vi "mobileye_decoder_PC.vi"(8 "can cluster":T1 {"identifier" format="%03x"}, 11 "name":string="Mobileye560") -> ()   [LabVIEW 2015]
uses:
  G_SEN.vi
  G_ALL.vi
panel:
  out "lane both":bool
  out "lane_left":dbl[](array[numeric])
  out "lane_right":dbl[](array[numeric])
  out "next lane left":dbl[][](array[numeric])
  out "next lane right":dbl[][](array[numeric])
  out "obs_tmp":dbl[][](array[numeric])
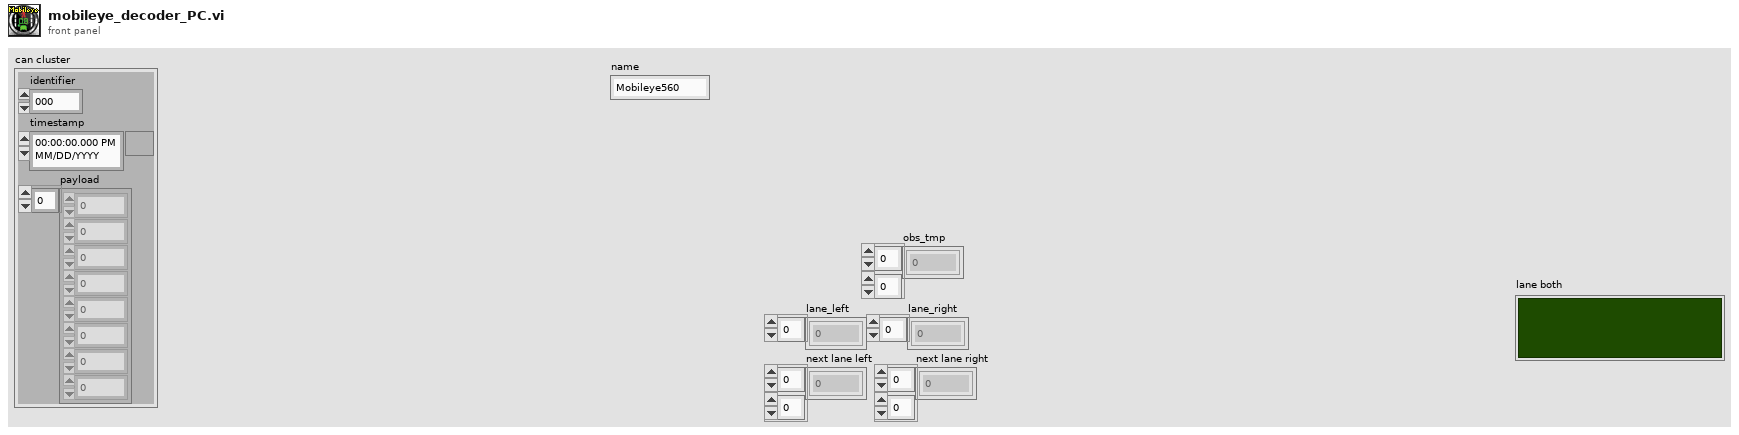
[diagram p1: front panel]
types:
  T1 = cluster{"identifier":u32, "timestamp":timestamp, "payload":u8[]}
  T2 = cluster{"C_Wheel base":dbl, "ratio_steer":dbl, "Overall width":dbl, "af":dbl, "turn radius":dbl, "eval":dbl, "ap":dbl, "an":dbl, "Vmax":dbl, "mu":dbl, "Vlast":dbl}
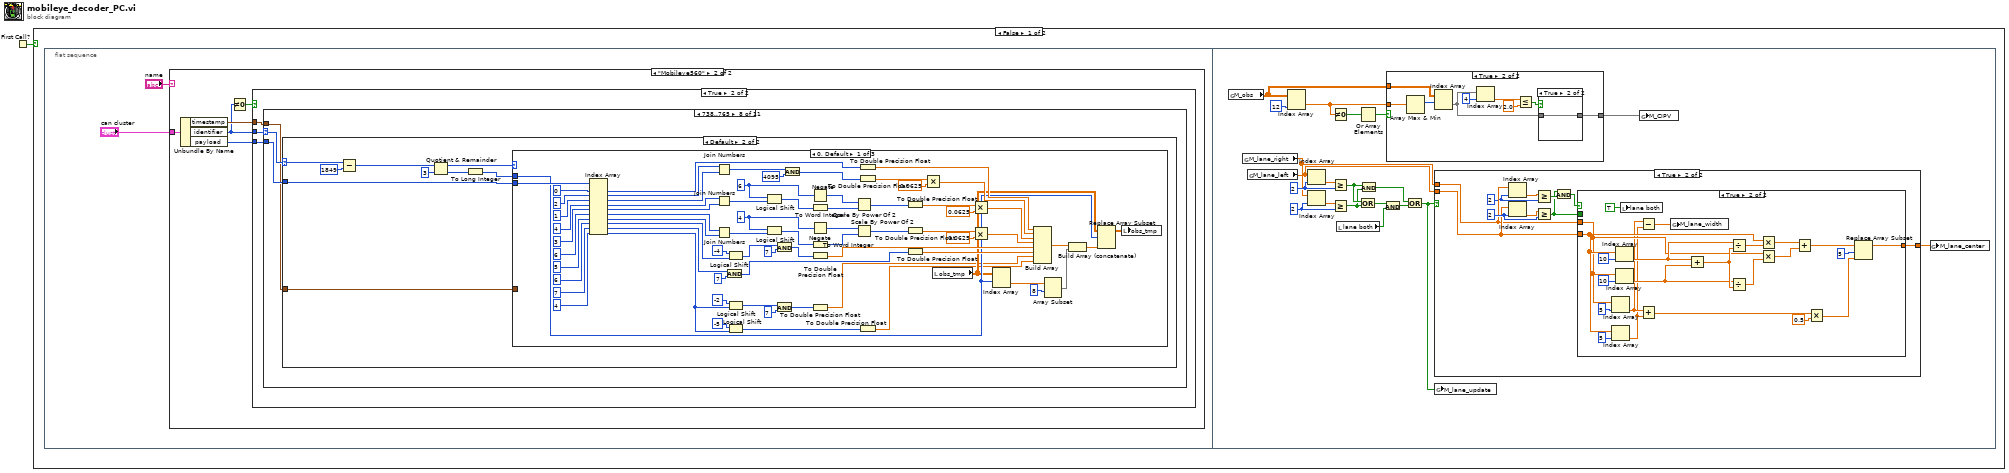
[diagram p0: block diagram]
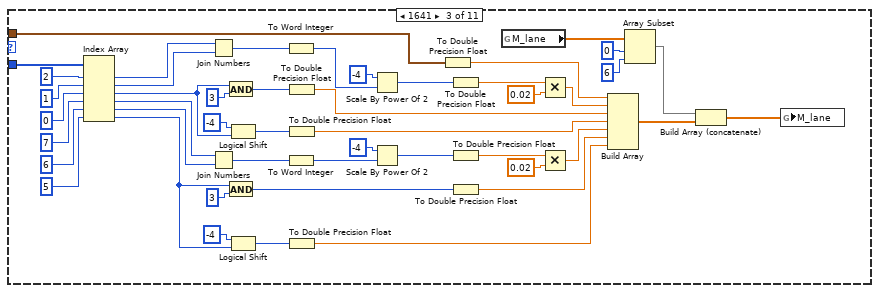
[diagram p6: hidden frame]
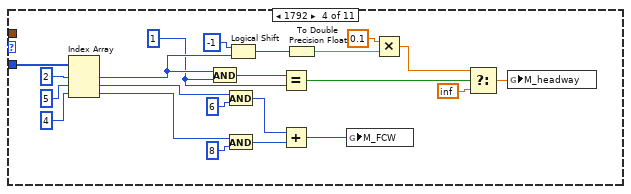
[diagram p7: hidden frame]
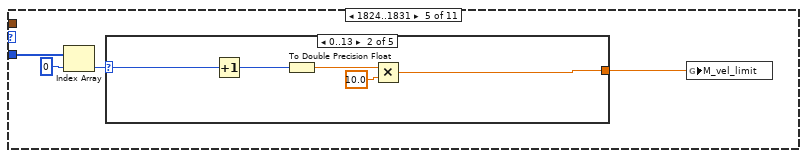
[diagram p8: hidden frame]
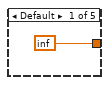
[diagram p9: hidden frame]
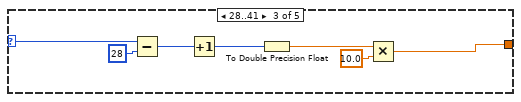
[diagram p10: hidden frame]
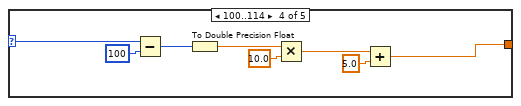
[diagram p11: hidden frame]
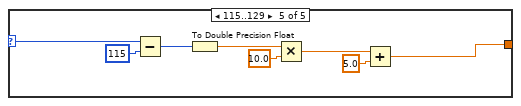
[diagram p12: hidden frame]
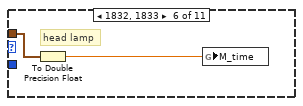
[diagram p13: hidden frame]
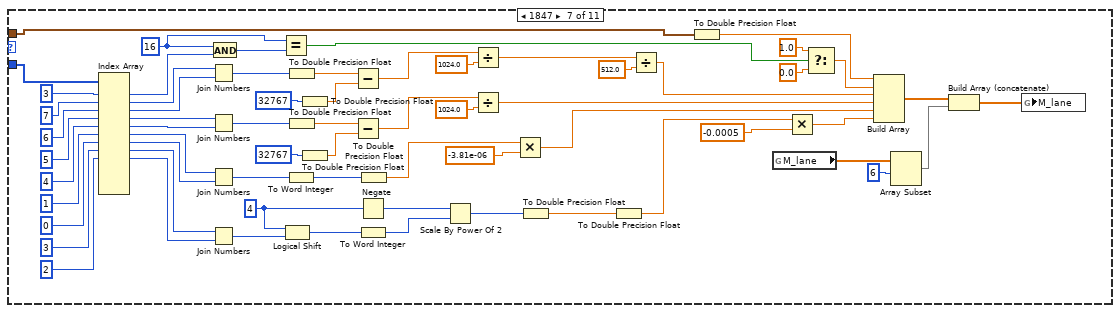
[diagram p14: hidden frame]
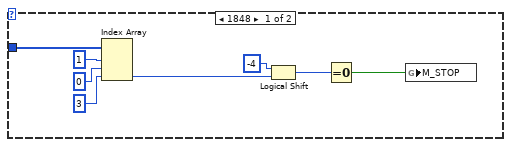
[diagram p15: hidden frame]
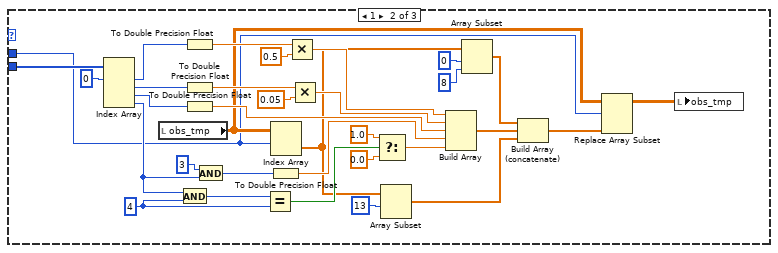
[diagram p16: hidden frame]
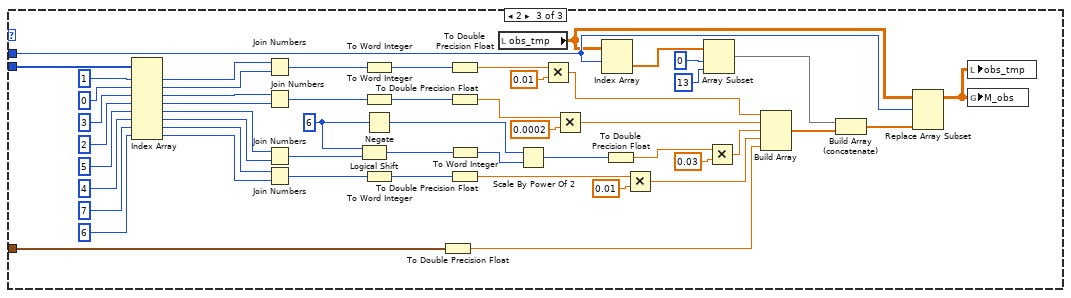
[diagram p17: hidden frame]
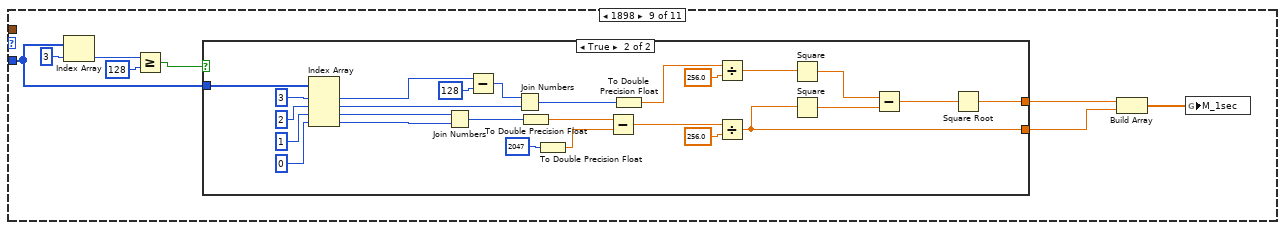
[diagram p18: hidden frame]
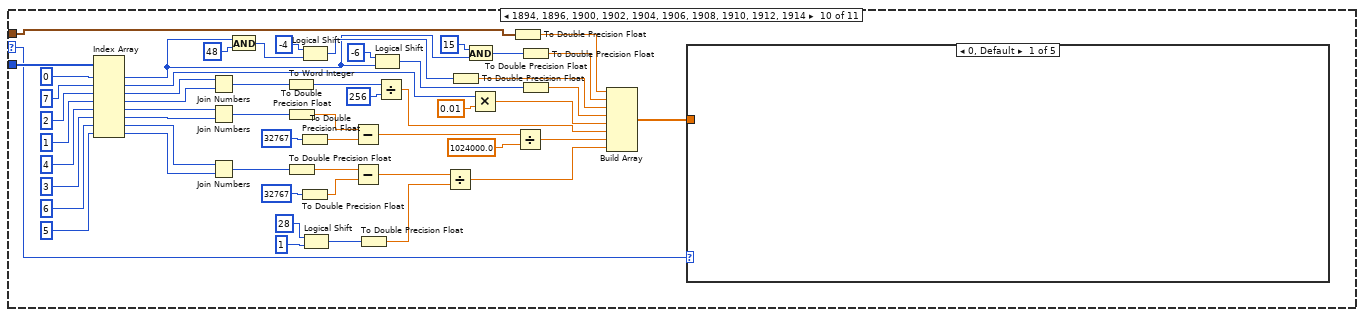
[diagram p20: hidden frame]
diagram:
  n1 = First Call?() -> (First Call?: T/F=w1:bool)
  n2 = case shown="False" w1 {
    frame False {
      n3 = flat-sequence {
        frame #0 {
          n4 = case shown="\"Mobileye560\"" "name" {
            tunnel: "can cluster" -> [_ w8]
            frame "False", Default {
            }
            frame "Mobileye560" {
              n5 = Unbundle By Name(w8) -> ("timestamp"=w6:timestamp, "identifier"=w5:u32, "payload"=w7:u8[])
              n6 = Not Equal To 0?(x=w5) -> (x != 0?=w4:bool)
              n7 = case shown="True" w4 {
                tunnel: w7 -> [_ w11]
                tunnel: w6 -> [_ w10]
                tunnel: w5 -> [_ w9]
                frame False {
                }
                frame True {
                  n8 = case shown="738..765" w9 {
                    selector: w9 -> [_ _ _ _ _ _ _ w181 _ w388 w469]
                    tunnel: w11 -> [_ _ w58 w80 w84 _ w178 w180 w357 w442 w497]
                    tunnel: w10 -> [_ _ w35 _ _ w115 w122 w179 _ w408 w472]
                    frame 0, Default {
                    }
                    frame 1616 {
                      # "Fixed Yaw horizontal"
                    }
                    frame 1641 {
                      n9 = Index Array(array=w58, index #1=2 ("index"), index #2=1 ("index"), index #3=0 ("index"), index #4=7 ("index"), index #5=6 ("index"), index #6=5 ("index")) -> (element #1=w55:u8, element #2=w54:u8, element #3=w33:u8, element #4=w26:u8, element #5=w25:u8, element #6=w21:u8)
                      n10 = Join Numbers(hi=w55, lo=w54) -> ((hi.lo)=w53:u16)
                      n11 = Join Numbers(hi=w26, lo=w25) -> ((hi.lo)=w48:u16)
                      n12 = And(x=w33, y=u8 3) -> (x .and. y?=w32:u8)
                      n13 = And(x=w21, y=u8 3) -> (x .and. y?=w24:u8)
                      n14 = Logical Shift(y=i16 -4, x=w33) -> (x << y=w31:u8)
                      n15 = Logical Shift(y=i16 -4, x=w21) -> (x << y=w28:u8)
                      n16 = To Word Integer(number=w53) -> (16bit integer=w40:i16)
                      n17 = To Word Integer(number=w48) -> (16bit integer=w37:i16)
                      n18 = To Double Precision Float(number=w32) -> (double precision float=w30:dbl)
                      n19 = To Double Precision Float(number=w31) -> (double precision float=w29:dbl)
                      n20 = To Double Precision Float(number=w28) -> (double precision float=w22:dbl)
                      n21 = Scale By Power Of 2(n=i16 -4 ("y"), x=w40) -> (x*2^n=w39:i16)
                      n22 = Scale By Power Of 2(n=i16 -4 ("y"), x=w37) -> (x*2^n=w36:i16)
                      n23 = To Double Precision Float(number=w35) -> (double precision float=w20:dbl)
                      n24 = To Double Precision Float(number=w39) -> (double precision float=w52:dbl)
                      n25 = To Double Precision Float(number=w36) -> (double precision float=w49:dbl)
                      n26 = To Double Precision Float(number=w24) -> (double precision float=w23:dbl)
                      n27 = global read "G_SEN.vi" "M_lane"() -> (w12:dbl[])
                      n28 = Multiply(x=w52, y=0.02) -> (x*y=w15:dbl)
                      n29 = Multiply(x=w49, y=0.02) -> (x*y=w14:dbl)
                      n30 = Build Array(w20, w15, w30, w29, w14, w23, w22) -> (w16:dbl[])
                      n31 = Array Subset(array=w12, index=0, length=6) -> (w17:dbl[])
                      n32 = Build Array (concatenate)(w17, w16) -> (w13:dbl[])
                      n33 = global write "G_SEN.vi" "M_lane"(w13) -> ()
                    }
                    frame 1792 {
                      w75 = u8 1 ("y")
                      n34 = Index Array(array=w80, index #1=2 ("index"), index #2=5 ("index"), index #3=4 ("index")) -> (element #1=w78:u8, element #2=w67:u8, element #3=w63:u8)
                      n35 = And(x=w78, y=w75) -> (x .and. y?=w76:u8)
                      n36 = And(x=w67, y=u8 6) -> (x .and. y?=w62:u8)
                      n37 = And(x=w63, y=u8 8) -> (x .and. y?=w61:u8)
                      n38 = Logical Shift(y=i16 -1, x=w78) -> (x << y=w73:u8)
                      n39 = Equal?(x=w76, y=w75) -> (x = y?=w74:bool)
                      n40 = Add(x=w62, y=w61) -> (x+y=w60:u8)
                      n41 = To Double Precision Float(number=w73) -> (double precision float=w72:dbl)
                      n42 = global write "G_SEN.vi" "M_FCW"(w60) -> ()
                      n43 = Multiply(x=0.1, y=w72) -> (x*y=w70:dbl)
                      n44 = Select(t=w70, s=w74, f=inf) -> (s? t:f=w59:dbl)
                      n45 = global write "G_SEN.vi" "M_headway"(w59) -> ()
                    }
                    frame 1824..1831 {
                      n46 = Index Array(array=w84, index=0) -> (element=w82:u8)
                      n47 = case shown="0..13" w82 {
                        selector: w82 -> [_ w90 w93 w103 w111]
                        tunnel: [inf w86 w94 w98 w106] -> w81
                        frame Default {
                        }
                        frame 0..13 {
                          n48 = Increment(x=w90) -> (x+1=w89:u8)
                          n49 = To Double Precision Float(number=w89) -> (double precision float=w88:dbl)
                          n50 = Multiply(x=w88, y=10.0) -> (x*y=w86:dbl)
                        }
                        frame 28..41 {
                          n51 = Subtract(x=w93, y=u8 28) -> (x-y=w92:u8)
                          n52 = Increment(x=w92) -> (x+1=w97:u8)
                          n53 = To Double Precision Float(number=w97) -> (double precision float=w96:dbl)
                          n54 = Multiply(x=w96, y=10.0) -> (x*y=w94:dbl)
                        }
                        frame 100..114 {
                          n55 = Subtract(x=w103, y=u8 100) -> (x-y=w101:u8)
                          n56 = To Double Precision Float(number=w101) -> (double precision float=w105:dbl)
                          n57 = Multiply(x=w105, y=10.0) -> (x*y=w100:dbl)
                          n58 = Add(x=w100, y=5.0) -> (x+y=w98:dbl)
                        }
                        frame 115..129 {
                          n59 = Subtract(x=w111, y=u8 115) -> (x-y=w109:u8)
                          n60 = To Double Precision Float(number=w109) -> (double precision float=w113:dbl)
                          n61 = Multiply(x=w113, y=10.0) -> (x*y=w108:dbl)
                          n62 = Add(x=w108, y=5.0) -> (x+y=w106:dbl)
                        }
                      }
                      n63 = global write "G_SEN.vi" "M_vel_limit"(w81) -> ()
                    }
                    frame 1832, 1833 {
                      # "head lamp"
                      n64 = To Double Precision Float(number=w115) -> (double precision float=w114:dbl)
                      n65 = global write "G_SEN.vi" "M_time"(w114) -> ()
                    }
                    frame 1847 {
                      w155 = u8 16 ("x")
                      w157 = i16 4 ("x")
                      n66 = Index Array(array=w178, index #1=3 ("index"), index #2=7 ("index"), index #3=6 ("index"), index #4=5 ("index"), index #5=4 ("index"), index #6=1 ("index"), index #7=0 ("index"), index #8=3 ("index"), index #9=2 ("index")) -> (element #1=w138:u8, element #2=w132:u8, element #3=w131:u8, element #4=w130:u8, element #5=w129:u8, element #6=w175:u8, element #7=w174:u8, element #8=w167:u8, element #9=w166:u8)  [unwired: 4 in, 4 out]
                      n67 = Join Numbers(hi=w132, lo=w131) -> ((hi.lo)=w154:u16)
                      n68 = Join Numbers(hi=w130, lo=w129) -> ((hi.lo)=w142:u16)
                      n69 = Join Numbers(hi=w175, lo=w174) -> ((hi.lo)=w173:u16)
                      n70 = Join Numbers(hi=w167, lo=w166) -> ((hi.lo)=w161:u16)
                      n71 = And(x=w155, y=w138) -> (x .and. y?=w156:u8)
                      n72 = Equal?(x=w155, y=w156) -> (x = y?=w141:bool)
                      n73 = Logical Shift(y=w157, x=w161) -> (x << y=w165:u16)
                      n74 = To Word Integer(number=w173) -> (16bit integer=w172:i16)
                      n75 = To Double Precision Float(number=w154) -> (double precision float=w153:dbl)
                      n76 = To Double Precision Float(number=w142) -> (double precision float=w143:dbl)
                      n77 = To Double Precision Float(number=i16 32767) -> (double precision float=w151:dbl)
                      n78 = To Double Precision Float(number=i16 32767) -> (double precision float=w145:dbl)
                      n79 = Subtract(x=w153, y=w151) -> (x-y=w150:dbl)
                      n80 = Subtract(x=w143, y=w145) -> (x-y=w146:dbl)
                      n81 = Negate(x=w157) -> (-x=w160:i16)
                      n82 = To Word Integer(number=w165) -> (16bit integer=w159:i16)
                      n83 = To Double Precision Float(number=w172) -> (double precision float=w171:dbl)
                      n84 = Scale By Power Of 2(n=w160, x=w159) -> (x*2^n=w158:i16)
                      n85 = Divide(x=w150, y=1024.0) -> (x/y=w127:dbl)
                      n86 = Divide(x=w146, y=1024.0) -> (x/y=w125:dbl)
                      n87 = Multiply(x=w171, y=-3.81e-06) -> (x*y=w124:dbl)
                      n88 = To Double Precision Float(number=w158) -> (double precision float=w162:dbl)
                      n89 = To Double Precision Float(number=w162) -> (double precision float=w163:dbl)
                      n90 = Divide(x=w127, y=512.0) -> (x/y=w126:dbl)
                      n91 = To Double Precision Float(number=w122) -> (double precision float=w118:dbl)
                      n92 = global read "G_SEN.vi" "M_lane"() -> (w116:dbl[])
                      n93 = Multiply(x=w163, y=-0.0005) -> (x*y=w123:dbl)
                      n94 = Select(t=1.0, s=w141, f=0.0) -> (s? t:f=w128:dbl)
                      n95 = Build Array(w118, w128, w126, w125, w124, w123) -> (w120:dbl[])
                      n96 = Array Subset(array=w116, index=6) -> (w119:dbl[])  [unwired: 1 in]
                      n97 = Build Array (concatenate)(w120, w119) -> (w117:dbl[])
                      n98 = global write "G_SEN.vi" "M_lane"(w117) -> ()
                    }
                    frame 1848..1893 {
                      n99 = case shown="Default" w181 {
                        selector: w181 -> [_ w194]
                        tunnel: w180 -> [w189 w193]
                        tunnel: w179 -> [_ w190]
                        frame 1848 {
                          n100 = Index Array(array=w189, index #1=1 ("index"), index #2=0 ("index"), index #3=3 ("index")) -> (element #3=w184:u8)  [unwired: 2 out]
                          n101 = Logical Shift(y=i16 -4, x=w184) -> (x << y=w186:u8)
                          n102 = Equal To 0?(x=w186) -> (x = 0?=w182:bool)
                          n103 = global write "G_SEN.vi" "M_STOP"(w182) -> ()
                        }
                        frame Default {
                          n104 = Subtract(x=w194, y=u32 1849) -> (x-y=w197:u32)
                          n105 = Quotient & Remainder(x=w197, y=u32 3) -> (x-y*floor(x/y)=w195:u32, floor(x/y)=w192:u32)
                          n106 = To Long Integer(number=w192) -> (32bit integer=w191:i32)
                          n107 = case shown="0, Default" w195 {
                            tunnel: w193 -> [w268 w301 w353]
                            tunnel: w191 -> [w222 w276 w352]
                            tunnel: w190 -> [_ _ w304]
                            frame 0, Default {
                              w211 = i16 4 ("y")
                              w215 = i16 6 ("y")
                              n108 = Index Array(array=w268, index #1=0 ("index"), index #2=2 ("index"), index #3=1 ("index"), index #4=4 ("index"), index #5=3 ("index"), index #6=6 ("index"), index #7=5 ("index"), index #8=6 ("index"), index #9=7 ("index"), index #10=4 ("index")) -> (element #1=w260:u8, element #2=w264:u8, element #3=w263:u8, element #4=w252:u8, element #5=w251:u8, element #6=w239:u8, element #7=w238:u8, element #8=w234:u8, element #9=w227:u8, element #10=w201:u8)
                              n109 = Join Numbers(hi=w264, lo=w263) -> ((hi.lo)=w255:u16)
                              n110 = Join Numbers(hi=w252, lo=w251) -> ((hi.lo)=w250:u16)
                              n111 = Join Numbers(hi=w239, lo=w238) -> ((hi.lo)=w240:u16)
                              n112 = And(x=w227, y=u8 7) -> (x .and. y?=w226:u8)
                              n113 = Logical Shift(y=i16 -4, x=w234) -> (x << y=w233:u8)
                              n114 = Logical Shift(y=i16 -2, x=w201) -> (x << y=w203:u8)
                              n115 = Logical Shift(y=i16 -5, x=w201) -> (x << y=w207:u8)
                              n116 = Logical Shift(y=w215, x=w250) -> (x << y=w249:u16)
                              n117 = Logical Shift(y=w211, x=w240) -> (x << y=w241:u16)
                              n118 = And(x=w233, y=u8 7) -> (x .and. y?=w231:u8)
                              n119 = And(x=w203, y=u8 7) -> (x .and. y?=w205:u8)
                              n120 = And(x=w255, y=u16 4095) -> (x .and. y?=w261:u16)
                              n121 = Negate(x=w215) -> (-x=w216:i16)
                              n122 = To Word Integer(number=w249) -> (16bit integer=w214:i16)
                              n123 = Negate(x=w211) -> (-x=w212:i16)
                              n124 = To Word Integer(number=w241) -> (16bit integer=w210:i16)
                              n125 = To Double Precision Float(number=w231) -> (double precision float=w230:dbl)
                              n126 = To Double Precision Float(number=w205) -> (double precision float=w200:dbl)
                              n127 = Scale By Power Of 2(n=w216, x=w214) -> (x*2^n=w213:i16)
                              n128 = Scale By Power Of 2(n=w212, x=w210) -> (x*2^n=w209:i16)
                              n129 = To Double Precision Float(number=w260) -> (double precision float=w257:dbl)
                              n130 = To Double Precision Float(number=w261) -> (double precision float=w259:dbl)
                              n131 = To Double Precision Float(number=w207) -> (double precision float=w199:dbl)
                              n132 = To Double Precision Float(number=w213) -> (double precision float=w246:dbl)
                              n133 = To Double Precision Float(number=w209) -> (double precision float=w243:dbl)
                              n134 = To Double Precision Float(number=w226) -> (double precision float=w225:dbl)
                              n135 = Multiply(x=w259, y=0.0625) -> (x*y=w256:dbl)
                              n136 = local read "obs_tmp"() -> (w221:dbl[][])
                              n137 = Multiply(x=w246, y=0.0625) -> (x*y=w247:dbl)
                              n138 = Multiply(x=w243, y=0.0625) -> (x*y=w237:dbl)
                              n139 = Index Array(array=w221, index (row)=w222) -> (element=w219:dbl[])  [unwired: 1 in]
                              n140 = Build Array(w257, w256, w247, w237, w230, w225, w200, w199) -> (w224:dbl[])
                              n141 = Array Subset(array=w219, index=8) -> (w218:dbl[])  [unwired: 1 in]
                              n142 = Build Array (concatenate)(w224, w218) -> (w223:dbl[])
                              n143 = Replace Array Subset(array=w221, new element=w223, index (row)=w222) -> (w220:dbl[][])  [unwired: 1 in]
                              n144 = local write "obs_tmp"(w220) -> ()
                            }
                            frame 1 {
                              w286 = u8 4 ("y")
                              n145 = Index Array(array=w301, index #1=0 ("index")) -> (element #1=w299:u8, element #2=w293:u8, element #3=w291:u8, element #4=w280:u8)  [unwired: 3 in]
                              n146 = local read "obs_tmp"() -> (w278:dbl[][])
                              n147 = And(x=w280, y=w286) -> (x .and. y?=w287:u8)
                              n148 = To Double Precision Float(number=w299) -> (double precision float=w298:dbl)
                              n149 = To Double Precision Float(number=w293) -> (double precision float=w294:dbl)
                              n150 = To Double Precision Float(number=w291) -> (double precision float=w290:dbl)
                              n151 = And(x=u8 3 ("y"), y=w280) -> (x .and. y?=w289:u8)
                              n152 = Equal?(x=w287, y=w286) -> (x = y?=w285:bool)
                              n153 = Index Array(array=w278, index (row)=w276) -> (element=w273:dbl[])  [unwired: 1 in]
                              n154 = To Double Precision Float(number=w289) -> (double precision float=w288:dbl)
                              n155 = Multiply(x=w298, y=0.5) -> (x*y=w296:dbl)
                              n156 = Multiply(x=w294, y=0.05) -> (x*y=w292:dbl)
                              n157 = Select(t=1.0, s=w285, f=0.0) -> (s? t:f=w282:dbl)
                              n158 = Array Subset(array=w273, index=13) -> (w269:dbl[])  [unwired: 1 in]
                              n159 = Build Array(w296, w292, w290, w288, w282) -> (w270:dbl[])
                              n160 = Array Subset(array=w273, index=0, length=8) -> (w271:dbl[])
                              n161 = Build Array (concatenate)(w271, w270, w269) -> (w279:dbl[])
                              n162 = Replace Array Subset(array=w278, new element=w279, index (row)=w276) -> (w277:dbl[][])  [unwired: 1 in]
                              n163 = local write "obs_tmp"(w277) -> ()
                            }
                            frame 2 {
                              w326 = i16 6 ("y")
                              n164 = Index Array(array=w353, index #1=1 ("index"), index #2=0 ("index"), index #3=3 ("index"), index #4=2 ("index"), index #5=5 ("index"), index #6=4 ("index"), index #7=7 ("index"), index #8=6 ("index")) -> (element #1=w349:u8, element #2=w348:u8, element #3=w336:u8, element #4=w335:u8, element #5=w331:u8, element #6=w330:u8, element #7=w314:u8, element #8=w313:u8)
                              n165 = Join Numbers(hi=w349, lo=w348) -> ((hi.lo)=w347:u16)
                              n166 = Join Numbers(hi=w336, lo=w335) -> ((hi.lo)=w337:u16)
                              n167 = Join Numbers(hi=w331, lo=w330) -> ((hi.lo)=w329:u16)
                              n168 = Join Numbers(hi=w314, lo=w313) -> ((hi.lo)=w315:u16)
                              n169 = Logical Shift(y=w326, x=w329) -> (x << y=w328:u16)
                              n170 = To Word Integer(number=w347) -> (16bit integer=w346:i16)
                              n171 = To Word Integer(number=w337) -> (16bit integer=w338:i16)
                              n172 = Negate(x=w326) -> (-x=w327:i16)
                              n173 = To Word Integer(number=w315) -> (16bit integer=w316:i16)
                              n174 = To Double Precision Float(number=w304) -> (double precision float=w303:dbl)
                              n175 = To Double Precision Float(number=w346) -> (double precision float=w345:dbl)
                              n176 = To Double Precision Float(number=w338) -> (double precision float=w339:dbl)
                              n177 = To Word Integer(number=w328) -> (16bit integer=w325:i16)
                              n178 = To Double Precision Float(number=w316) -> (double precision float=w317:dbl)
                              n179 = local read "obs_tmp"() -> (w311:dbl[][])
                              n180 = Scale By Power Of 2(n=w327, x=w325) -> (x*2^n=w324:i16)
                              n181 = Multiply(x=w345, y=0.01) -> (x*y=w343:dbl)
                              n182 = Multiply(x=w339, y=0.0002) -> (x*y=w334:dbl)
                              n183 = Index Array(array=w311, index (row)=w352) -> (element=w308:dbl[])  [unwired: 1 in]
                              n184 = To Double Precision Float(number=w324) -> (double precision float=w322:dbl)
                              n185 = Multiply(x=w317, y=0.01) -> (x*y=w312:dbl)
                              n186 = Array Subset(array=w308, index=0, length=13) -> (w305:dbl[])
                              n187 = Multiply(x=w322, y=0.03) -> (x*y=w321:dbl)
                              n188 = Build Array(w343, w334, w321, w312, w303) -> (w307:dbl[])
                              n189 = Build Array (concatenate)(w305, w307) -> (w306:dbl[])
                              n190 = Replace Array Subset(array=w311, new element=w306, index (row)=w352) -> (w302:dbl[][])  [unwired: 1 in]
                              n191 = local write "obs_tmp"(w302) -> ()
                              n192 = global write "G_SEN.vi" "M_obs"(w302) -> ()
                            }
                          }
                        }
                      }
                    }
                    frame 1898 {
                      n193 = Index Array(array=w357, index=3) -> (element=w360:u8)
                      n194 = Greater Or Equal?(x=w360, y=u8 128) -> (x >= y?=w358:bool)
                      n195 = case shown="True" w358 {
                        tunnel: w357 -> [_ w387]
                        tunnel: [_ w362] -> w356
                        tunnel: [_ w364] -> w355
                        frame False {
                        }
                        frame True {
                          n196 = Index Array(array=w387, index #1=3 ("index"), index #2=2 ("index"), index #3=1 ("index"), index #4=0 ("index")) -> (element #1=w378:u8, element #2=w382:u8, element #3=w381:u8, element #4=w380:u8)
                          n197 = Join Numbers(hi=w381, lo=w380) -> ((hi.lo)=w368:u16)
                          n198 = Subtract(x=w378, y=u8 128) -> (x-y=w377:u8)
                          n199 = Join Numbers(hi=w377, lo=w382) -> ((hi.lo)=w370:u16)
                          n200 = To Double Precision Float(number=w368) -> (double precision float=w376:dbl)
                          n201 = To Double Precision Float(number=u16 2047 ("(hi.lo)")) -> (double precision float=w375:dbl)
                          n202 = Subtract(x=w376, y=w375) -> (x-y=w373:dbl)
                          n203 = To Double Precision Float(number=w370) -> (double precision float=w369:dbl)
                          n204 = Divide(x=w369, y=256.0) -> (x/y=w367:dbl)
                          n205 = Divide(x=w373, y=256.0) -> (x/y=w364:dbl)
                          n206 = Square(x=w367) -> (x^2=w366:dbl)
                          n207 = Square(x=w364) -> (x^2=w365:dbl)
                          n208 = Subtract(x=w366, y=w365) -> (x-y=w363:dbl)
                          n209 = Square Root(x=w363) -> (sqrt(x)=w362:dbl)
                        }
                      }
                      n210 = Build Array(w356, w355) -> (w354:dbl[])
                      n211 = global write "G_SEN.vi" "M_1sec"(w354) -> ()
                    }
                    frame 1894, 1896, 1900, 1902, 1904, 1906, 1908, 1910, 1912, 1914 {
                      n212 = Index Array(array=w442, index #1=0 ("index"), index #2=7 ("index"), index #3=2 ("index"), index #4=1 ("index"), index #5=4 ("index"), index #6=3 ("index"), index #7=6 ("index"), index #8=5 ("index")) -> (element #1=w398:u8, element #2=w393:u8, element #3=w440:u8, element #4=w439:u8, element #5=w432:u8, element #6=w431:u8, element #7=w422:u8, element #8=w421:u8)
                      n213 = Join Numbers(hi=w440, lo=w439) -> ((hi.lo)=w438:u16)
                      n214 = Join Numbers(hi=w432, lo=w431) -> ((hi.lo)=w430:u16)
                      n215 = Join Numbers(hi=w422, lo=w421) -> ((hi.lo)=w415:u16)
                      n216 = And(x=w398, y=u8 48) -> (x .and. y?=w403:u8)
                      n217 = To Word Integer(number=w438) -> (16bit integer=w437:i16)
                      n218 = To Double Precision Float(number=w430) -> (double precision float=w427:dbl)
                      n219 = To Double Precision Float(number=w415) -> (double precision float=w418:dbl)
                      n220 = Logical Shift(y=i16 -4, x=w403) -> (x << y=w401:u8)
                      n221 = To Double Precision Float(number=u16 32767 ("y")) -> (double precision float=w428:dbl)
                      n222 = To Double Precision Float(number=u16 32767 ("y")) -> (double precision float=w417:dbl)
                      n223 = Logical Shift(y=28, x=1) -> (x << y=w412:i32)
                      n224 = Subtract(x=w427, y=w428) -> (x-y=w426:dbl)
                      n225 = Subtract(x=w418, y=w417) -> (x-y=w410:dbl)
                      n226 = To Double Precision Float(number=w412) -> (double precision float=w411:dbl)
                      n227 = Logical Shift(y=i16 -6, x=w398) -> (x << y=w396:u8)
                      n228 = Divide(x=w437, y=i16 256) -> (x/y=w423:dbl)
                      n229 = Divide(x=w410, y=w411) -> (x/y=w409:dbl)
                      n230 = To Double Precision Float(number=w401) -> (double precision float=w399:dbl)
                      n231 = And(x=u8 15, y=w398) -> (x .and. y?=w405:u8)
                      n232 = Multiply(x=w393, y=0.01) -> (x*y=w391:dbl)
                      n233 = To Double Precision Float(number=w408) -> (double precision float=w390:dbl)
                      n234 = Divide(x=w426, y=1024000.0) -> (x/y=w424:dbl)
                      n235 = To Double Precision Float(number=w405) -> (double precision float=w400:dbl)
                      n236 = To Double Precision Float(number=w396) -> (double precision float=w395:dbl)
                      n237 = Build Array(w390, w400, w399, w395, w391, w423, w424, w409) -> (w389:dbl[])
                      n238 = case shown="0, Default" w388 {
                        selector: w388 -> [_ _ _ w458 w466]
                        tunnel: w389 -> [_ w444 w450 w459 w467]
                        frame 0, Default {
                        }
                        frame 1894 {
                          n239 = local read "lane_left"() -> (w447:dbl[])
                          n240 = Array Subset(array=w447, index=8) -> (w445:dbl[])  [unwired: 1 in]
                          n241 = Build Array (concatenate)(w444, w445) -> (w443:dbl[])
                          n242 = local write "lane_left"(w443) -> ()
                        }
                        frame 1896 {
                          n243 = local read "lane_right"() -> (w452:dbl[])
                          n244 = Array Subset(array=w452, index=8) -> (w449:dbl[])  [unwired: 1 in]
                          n245 = Build Array (concatenate)(w450, w449) -> (w448:dbl[])
                          n246 = local write "lane_right"(w448) -> ()
                        }
                        frame 1900, 1904, 1908, 1912 {
                          n247 = Subtract(x=w458, y=u32 1900) -> (x-y=w456:u32)
                          n248 = Quotient & Remainder(x=w456, y=u32 4) -> (floor(x/y)=w454:u32)  [unwired: 1 out]
                          n249 = local read "next lane left"() -> (w460:dbl[][])
                          n250 = Replace Array Subset(array=w460, new element=w459, index (row)=w454) -> (w453:dbl[][])  [unwired: 1 in]
                          n251 = local write "next lane left"(w453) -> ()
                        }
                        frame 1902, 1906, 1910, 1914 {
                          n252 = Subtract(x=w466, y=u32 1900) -> (x-y=w464:u32)
                          n253 = Quotient & Remainder(x=w464, y=u32 4) -> (floor(x/y)=w462:u32)  [unwired: 1 out]
                          n254 = local read "next lane right"() -> (w468:dbl[][])
                          n255 = Replace Array Subset(array=w468, new element=w467, index (row)=w462) -> (w461:dbl[][])  [unwired: 1 in]
                          n256 = local write "next lane right"(w461) -> ()
                        }
                      }
                    }
                    frame 1895, 1897, 1901, 1903, 1905, 1907, 1909, 1911, 1913, 1915 {
                      w479 = u16 32768 ("y")
                      n257 = Index Array(array=w497, index #1=1 ("index"), index #2=0 ("index"), index #3=3 ("index"), index #4=2 ("index")) -> (element #1=w494:u8, element #2=w493:u8, element #3=w484:u8, element #4=w483:u8)
                      n258 = Join Numbers(hi=w494, lo=w493) -> ((hi.lo)=w489:u16)
                      n259 = Join Numbers(hi=w484, lo=w483) -> ((hi.lo)=w480:u16)
                      n260 = Subtract(x=w480, y=w479) -> (x-y=w478:u16)
                      n261 = And(x=w479, y=w480) -> (x .and. y?=w482:u16)
                      n262 = To Double Precision Float(number=w489) -> (double precision float=w490:dbl)
                      n263 = To Double Precision Float(number=u16 32767 ("y")) -> (double precision float=w491:dbl)
                      n264 = Subtract(x=w490, y=w491) -> (x-y=w488:dbl)
                      n265 = Equal?(x=w479, y=w482) -> (x = y?=w481:bool)
                      n266 = Divide(x=w478, y=u16 256) -> (x/y=w476:dbl)
                      n267 = Select(t=w476, s=w481, f=0.0) -> (s? t:f=w473:dbl)
                      n268 = Divide(x=w488, y=1024.0) -> (x/y=w474:dbl)
                      n269 = To Double Precision Float(number=w472) -> (double precision float=w471:dbl)
                      n270 = Build Array(w471, w474, w473) -> (w470:dbl[])
                      n271 = case shown="767" w469 {
                        selector: w469 -> [_ _ _ w519 w534]
                        tunnel: w470 -> [_ w499 w505 w515 w530]
                        frame 0, Default {
                        }
                        frame 1895 {
                          n272 = local read "lane_left"() -> (w503:dbl[])
                          n273 = Array Subset(array=w503, index=0, length=8 ("index")) -> (w502:dbl[])
                          n274 = Build Array (concatenate)(w502, w499) -> (w498:dbl[])
                          n275 = local write "lane_left"(w498) -> ()
                          n276 = global write "G_SEN.vi" "M_lane_left"(w498) -> ()
                        }
                        frame 1897 {
                          n277 = local read "lane_right"() -> (w509:dbl[])
                          n278 = Array Subset(array=w509, index=0, length=8 ("index")) -> (w508:dbl[])
                          n279 = Build Array (concatenate)(w508, w505) -> (w504:dbl[])
                          n280 = local write "lane_right"(w504) -> ()
                          n281 = global write "G_SEN.vi" "M_lane_right"(w504) -> ()
                        }
                        frame 1901, 1905, 1909, 1913 {
                          n282 = Subtract(x=w519, y=u32 1900) -> (x-y=w522:u32)
                          n283 = local read "next lane left"() -> (w524:dbl[][])
                          n284 = Quotient & Remainder(x=w522, y=u32 4) -> (floor(x/y)=w516:u32)  [unwired: 1 out]
                          n285 = Index Array(array=w515, index #1=0 ("index")) -> (element #1=w513:dbl, element #2=w512:dbl, element #3=w511:dbl)  [unwired: 2 in]
                          n286 = Replace Array Subset(array=w524, new element #1=w513, index (row) #1=w516, index (col) #1=8 ("disabled index (col)"), new element #2=w512, index (row) #2=w516, index (col) #2=9 ("disabled index (col)"), new element #3=w511, index (row) #3=w516, index (col) #3=10 ("index (col)")) -> (w510:dbl[][])
                          n287 = local write "next lane left"(w510) -> ()
                          n288 = global write "G_SEN.vi" "M_next lane left"(w510) -> ()
                        }
                        frame 1903, 1907, 1911, 1915 {
                          n289 = Subtract(x=w534, y=u32 1900) -> (x-y=w537:u32)
                          n290 = local read "next lane right"() -> (w539:dbl[][])
                          n291 = Quotient & Remainder(x=w537, y=u32 4) -> (floor(x/y)=w531:u32)  [unwired: 1 out]
                          n292 = Index Array(array=w530, index #1=0 ("index")) -> (element #1=w528:dbl, element #2=w527:dbl, element #3=w526:dbl)  [unwired: 2 in]
                          n293 = Replace Array Subset(array=w539, new element #1=w528, index (row) #1=w531, index (col) #1=8 ("disabled index (col)"), new element #2=w527, index (row) #2=w531, index (col) #2=9 ("disabled index (col)"), new element #3=w526, index (row) #3=w531, index (col) #3=10 ("index (col)")) -> (w525:dbl[][])
                          n294 = local write "next lane right"(w525) -> ()
                          n295 = global write "G_SEN.vi" "M_next lane right"(w525) -> ()
                        }
                      }
                    }
                  }
                }
              }
            }
          }
        }
        frame #1 {
          w551 = 2 ("index")
          w555 = 2 ("index")
          n296 = global read "G_SEN.vi" "M_obs"() -> (w541:dbl[][])
          n297 = global read "G_SEN.vi" "M_lane_right"() -> (w549:dbl[])
          n298 = global read "G_SEN.vi" "M_lane_left"() -> (w548:dbl[])
          n299 = Index Array(array=w541, index (col)=12 ("disabled index (col)")) -> (element=w542:dbl[])  [unwired: 1 in]
          n300 = Index Array(array=w548, index=w555) -> (element=w554:dbl)
          n301 = Index Array(array=w549, index=w551) -> (element=w552:dbl)
          n302 = Not Equal To 0?(x=w542) -> (x != 0?=w544:bool[])
          n303 = Greater Or Equal?(x=w554, y=w555) -> (x >= y?=w553:bool)
          n304 = Greater Or Equal?(x=w552, y=w551) -> (x >= y?=w550:bool)
          n305 = local read "lane both"() -> (w558:bool)
          n306 = Or(x=w553, y=w550) -> (x .or. y?=w559:bool)
          n307 = Or Array Elements(Boolean array=w544) -> (logical OR=w543:bool)
          n308 = And(x=w553, y=w550) -> (x .and. y?=w557:bool)
          n309 = And(x=w559, y=w558) -> (x .and. y?=w556:bool)
          n310 = case shown="True" w543 {
            tunnel: w542 -> [_ w568]
            tunnel: w541 -> [_ w567]
            tunnel: [_ w560] -> w540
            frame False {
            }
            frame True {
              n311 = Array Max & Min(array=w568) -> (max index (indices)=w566:i32)  [unwired: 3 out]
              n312 = Index Array(array=w567, index (row)=w566) -> (element=w565:dbl[])  [unwired: 1 in]
              n313 = Index Array(array=w565, index=4) -> (element=w563:dbl)
              n314 = Less Or Equal?(x=w563, y=2.0) -> (x <= y?=w561:bool)
              n315 = case shown="True" w561 {
                tunnel: w565 -> [_ w569]
                tunnel: [_ w569] -> w560
                frame False {
                }
                frame True {
                }
              }
            }
          }
          n316 = Or(x=w557, y=w556) -> (x .or. y?=w546:bool)
          n317 = case shown="True" w546 {
            tunnel: w548 -> [_ w574]
            tunnel: w549 -> [_ w573]
            tunnel: [_ w572] -> w547
            frame False {
            }
            frame True {
              w570 = 2 ("index")
              w579 = 2 ("index")
              n318 = Index Array(array=w573, index=w570) -> (element=w571:dbl)
              n319 = Index Array(array=w574, index=w579) -> (element=w578:dbl)
              n320 = Greater Or Equal?(x=w571, y=w570) -> (x >= y?=w577:bool)
              n321 = Greater Or Equal?(x=w578, y=w579) -> (x >= y?=w575:bool)
              n322 = And(x=w575, y=w577) -> (x .and. y?=w576:bool)
              n323 = case shown="True" w576 {
                tunnel: w574 -> [w602 w617]
                tunnel: w573 -> [w597 w613]
                tunnel: [w594 w603] -> w572
                tunnel: w575 -> [w596 _]
                frame False {
                  w589 = 0.2 ("y")
                  w592 = 5 ("index")
                  w601 = 5 ("index")
                  n324 = global read "G_ALL.vi" "CARSPEC"() -> (w581:T2)
                  n325 = Index Array(array=w602, index=w601) -> (element=w599:dbl)
                  n326 = Index Array(array=w597, index=w592) -> (element=w591:dbl)
                  n327 = Unbundle By Name(w581) -> ("Overall width"=w580:dbl)
                  n328 = global read "G_SEN.vi" "M_lane_width"() -> (w582:dbl)
                  n329 = Multiply(x=w580, y=w589) -> (x*y=w587:dbl)
                  n330 = Add(x=w587, y=w589) -> (x+y=w583:dbl)
                  n331 = Add(x=1.0 ("y"), y=w587) -> (x+y=w584:dbl)
                  n332 = Multiply(x=w582, y=0.5) -> (x*y=w586:dbl)
                  n333 = In Range and Coerce(upper limit=w584, x=w586, lower limit=w583) -> (coerced(x)=w585:dbl)  [unwired: 1 out]
                  n334 = Add(x=w599, y=w585) -> (x+y=w598:dbl)
                  n335 = Subtract(x=w591, y=w585) -> (x-y=w590:dbl)
                  n336 = Replace Array Subset(array=w602, new element=w598, index=w601) -> (w595:dbl[])
                  n337 = Replace Array Subset(array=w597, new element=w590, index=w592) -> (w593:dbl[])
                  n338 = Select(t=w595, s=w596, f=w593) -> (s? t:f=w594:dbl[])
                }
                frame True {
                  n339 = Index Array(array=w613, index=5) -> (element=w610:dbl)
                  n340 = Index Array(array=w617, index=5) -> (element=w609:dbl)
                  n341 = Index Array(array=w617, index=10) -> (element=w619:dbl)
                  n342 = Index Array(array=w613, index=10) -> (element=w614:dbl)
                  n343 = local write "lane both"(TRUE ("lane both")) -> ()
                  n344 = Subtract(x=w610, y=w609) -> (x-y=w622:dbl)
                  n345 = Add(x=w610, y=w609) -> (x+y=w608:dbl)
                  n346 = global write "G_SEN.vi" "M_lane_width"(w622) -> ()
                  n347 = Add(x=w619, y=w614) -> (x+y=w615:dbl)
                  n348 = Divide(x=w619, y=w615) -> (x/y=w618:dbl)
                  n349 = Divide(x=w614, y=w615) -> (x/y=w616:dbl)
                  n350 = Multiply(x=w617, y=w618) -> (x*y=w612:dbl[])
                  n351 = Multiply(x=w613, y=w616) -> (x*y=w611:dbl[])
                  n352 = Add(x=w612, y=w611) -> (x+y=w606:dbl[])
                  n353 = Multiply(x=w608, y=0.5) -> (x*y=w605:dbl)
                  n354 = Replace Array Subset(array=w606, new element=w605, index=5) -> (w603:dbl[])
                }
              }
            }
          }
          n355 = global write "G_SEN.vi" "M_lane_update"(w546) -> ()
          n356 = global write "G_SEN.vi" "M_CIPV"(w540) -> ()
          n357 = global write "G_SEN.vi" "M_lane_center"(w547) -> ()
        }
      }
    }
    frame True {
      n358 = global write "G_SEN.vi" "M_lane_width"(3.5 ("M_lane_width")) -> ()
      n359 = Initialize Array(0.0, 11 ("dimension size")) -> (→"lane_left" →"lane_right":dbl[])
      n360 = Initialize Array(0.0 ("element"), 64 ("dimension size"), 18 ("dimension size")) -> (→"obs_tmp":dbl[][])
      n361 = Initialize Array(0.0, 4 ("dimension size"), 11 ("dimension size")) -> (→"next lane left" →"next lane right":dbl[][])
      "lane both" <- FALSE ("lane both")
    }
  }
